vi "Coord window-Key press handler.vi"(4 "ScanCode":i16, 6 "Char":i16, 9 "VKey":T2, 11 "PlatMods":T1) -> ()   [LabVIEW 2020]
uses:
  <vilib>/event_ctls.llb/eventvkey.ctl
  Visualisation/Functional Imaging Viewer/SubVIs/Experiment header interface/Typedefs/Save-Load-Save as-Load last enum.ctl
  Globals/Coord window-Globals.vi
panel:
  out "error out":errorcluster
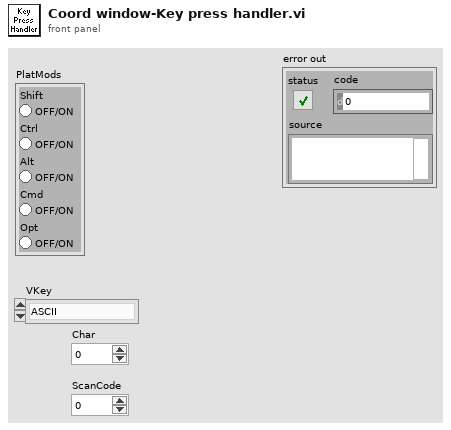
[diagram p1: front panel]
types:
  T1 = cluster{"Shift":bool, "Ctrl":bool, "Alt":bool, "Cmd":bool, "Opt":bool}
  T2 = typedef "eventvkey.ctl" = enum16{"ASCII", "Enter", "Return", "Shift", "Ctrl", "Alt", "Cmd", "Opt", "Caps", "NumLock", "Clear", "Break", "Up", "Down", "Left", "Right", "Insert", "Delete", "Home", "End", "PageUp", "PageDown", "Escape", "Help", "Pause", "ScrollLock", "F1", "F2", "F3", "F4", "F5", "F6", "F7", "F8", "F9", "F10", "F11", "F12", "F13", "F14", "F15", "F16", "F17", "F18", "F19", "F20", "F21", "F22", "F23", "F24", "Play", "VolumeUp", "VolumeDown", "Mute", "Two Byte Char"}
  T3 = typedef "Save-Load-Save as-Load last enum.ctl" = enum16{"Save file", "Save file as", "Load file", "Load last file"}
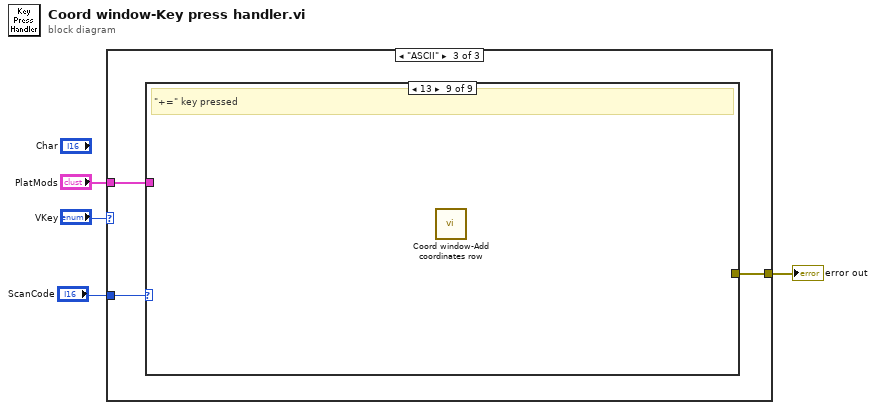
[diagram p0: block diagram]
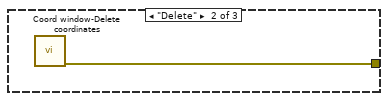
[diagram p3: hidden frame]
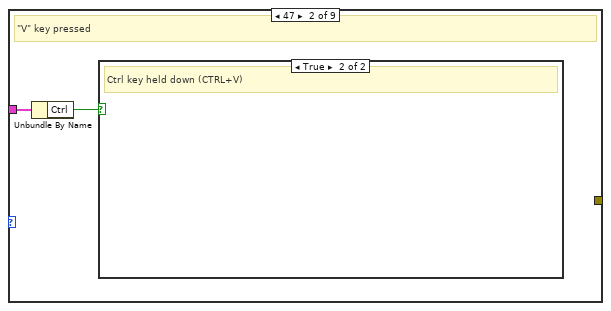
[diagram p5: hidden frame]
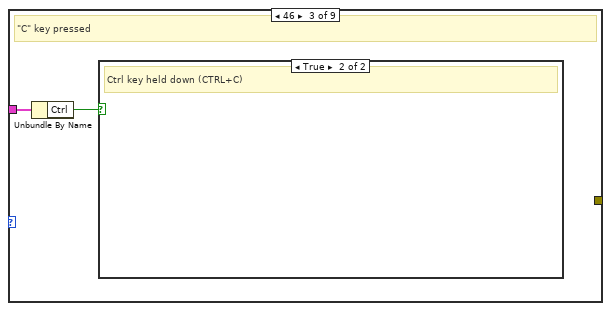
[diagram p7: hidden frame]
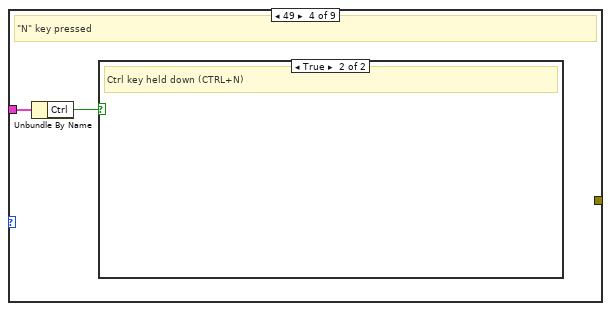
[diagram p9: hidden frame]
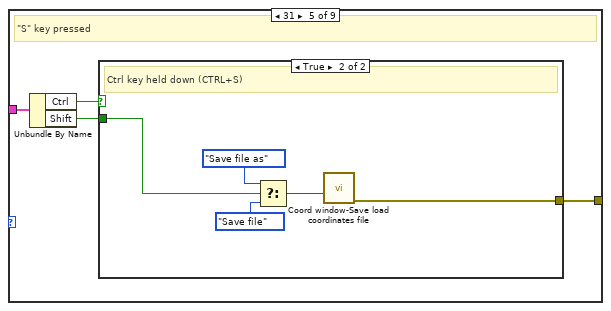
[diagram p11: hidden frame]
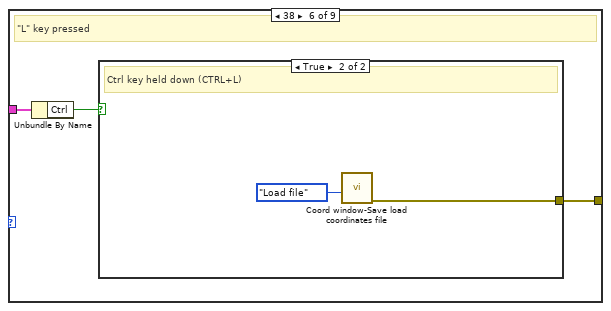
[diagram p13: hidden frame]
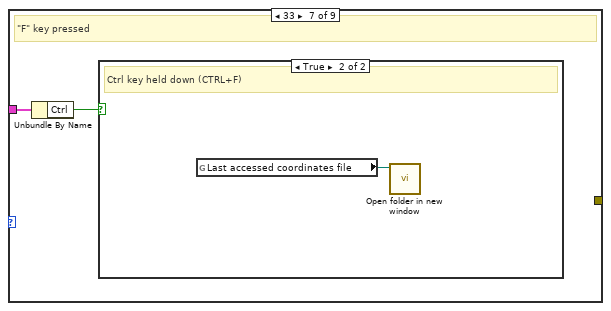
[diagram p15: hidden frame]
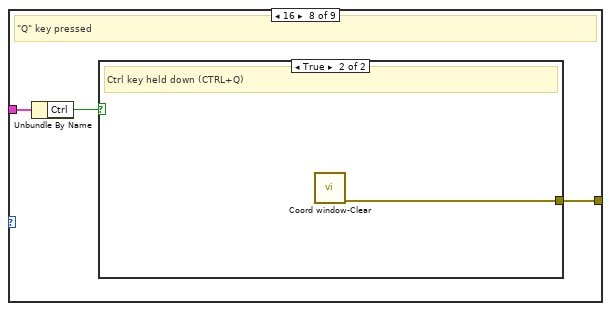
[diagram p17: hidden frame]
diagram:
  n1 = case shown="\"ASCII\"" "VKey" {
    tunnel: [_ w5 w7] -> w4
    tunnel: "PlatMods" -> [_ _ w8]
    tunnel: "ScanCode" -> [_ _ w6]
    frame Default {
    }
    frame "Delete" {
      n2 = call "Coord window-Delete coordinates.vi"() -> ("error out"=w5:errorcluster)  [unwired: 11 in]
    }
    frame "ASCII" {
      n3 = case shown="13" w6 {
        tunnel: w8 -> [_ w10 w12 w14 w18 w26 w30 w34 _]
        tunnel: [_ _ _ _ w16 w24 _ w32 _] -> w7
        frame Default {
        }
        frame 47 {
          # "\"V\" key pressed"
          n4 = Unbundle By Name(w10) -> ("Ctrl"=w9:bool)
          n5 = case shown="True" w9 {
            frame False {
            }
            frame True {
              # "Ctrl key held down (CTRL+V)"
            }
          }
        }
        frame 46 {
          # "\"C\" key pressed"
          n6 = Unbundle By Name(w12) -> ("Ctrl"=w11:bool)
          n7 = case shown="True" w11 {
            frame False {
            }
            frame True {
              # "Ctrl key held down (CTRL+C)"
            }
          }
        }
        frame 49 {
          # "\"N\" key pressed"
          n8 = Unbundle By Name(w14) -> ("Ctrl"=w13:bool)
          n9 = case shown="True" w13 {
            frame False {
            }
            frame True {
              # "Ctrl key held down (CTRL+N)"
            }
          }
        }
        frame 31 {
          # "\"S\" key pressed"
          n10 = Unbundle By Name(w18) -> ("Ctrl"=w17:bool, "Shift"=w15:bool)
          n11 = case shown="True" w17 {
            tunnel: [_ w23] -> w16
            tunnel: w15 -> [_ w22]
            frame False {
            }
            frame True {
              # "Ctrl key held down (CTRL+S)"
              n12 = Select(t=Save-Load-Save_as-Load_last_enum."Save file as" ("Function"), s=w22, f=Save-Load-Save_as-Load_last_enum."Save file" ("Function")) -> (s? t:f=w19:T3)
              n13 = call "Coord window-Save load coordinates file.vi"("Function"=w19) -> ("error out"=w23:errorcluster)  [unwired: 10 in]
            }
          }
        }
        frame 38 {
          # "\"L\" key pressed"
          n14 = Unbundle By Name(w26) -> ("Ctrl"=w25:bool)
          n15 = case shown="True" w25 {
            tunnel: [_ w27] -> w24
            frame False {
            }
            frame True {
              # "Ctrl key held down (CTRL+L)"
              n16 = call "Coord window-Save load coordinates file.vi"("Function"=Save-Load-Save_as-Load_last_enum."Load file") -> ("error out"=w27:errorcluster)  [unwired: 10 in]
            }
          }
        }
        frame 33 {
          # "\"F\" key pressed"
          n17 = Unbundle By Name(w30) -> ("Ctrl"=w29:bool)
          n18 = case shown="True" w29 {
            frame False {
            }
            frame True {
              # "Ctrl key held down (CTRL+F)"
              n19 = global read "Coord window-Globals.vi" "Last accessed coordinates file"() -> (w31:path)
              n20 = call "Open folder in new window.vi"("Directory to open"=w31) -> ()  [unwired: 10 in, 1 out]
            }
          }
        }
        frame 16 {
          # "\"Q\" key pressed"
          n21 = Unbundle By Name(w34) -> ("Ctrl"=w33:bool)
          n22 = case shown="True" w33 {
            tunnel: [_ w35] -> w32
            frame False {
            }
            frame True {
              # "Ctrl key held down (CTRL+Q)"
              n23 = call "Coord window-Clear.vi"() -> ("error out"=w35:errorcluster)  [unwired: 11 in]
            }
          }
        }
        frame 13 {
          # "\"+=\" key pressed"
          n24 = call "Coord window-Add coordinates row.vi"() -> ()  [unwired: 11 in, 1 out]
        }
      }
    }
  }
  "error out" <- w4
